vi "Read.vi"(7 "timeout (100ms)":i32=100, 8 "error in (no error)":errorcluster, 9 "Interlock in":bool, 11 "Interlock Bool in":refnum<class "Interlock Bool.lvclass">) -> (0 "error out":errorcluster, 1 "Interlock":bool, 2 "Data out":variant, 3 "Interlock Bool out":refnum<class "Interlock Bool.lvclass">, 4 "IL Action":refnum<class "IL Action.lvclass">[](array[class]))   [LabVIEW 2015, in "Interlocks.lvlib" / "Interlock Bool.lvclass"]
uses:
  Interlock Bool.lvclass
  IL Action/IL Action.lvclass
  Interlock/State Enum.ctl
  Interlock Bool.lvclass/Interlock Bool.ctl
  Interlock/Interlock.lvclass/Interlock.ctl
  Interlock/Interlock.lvclass
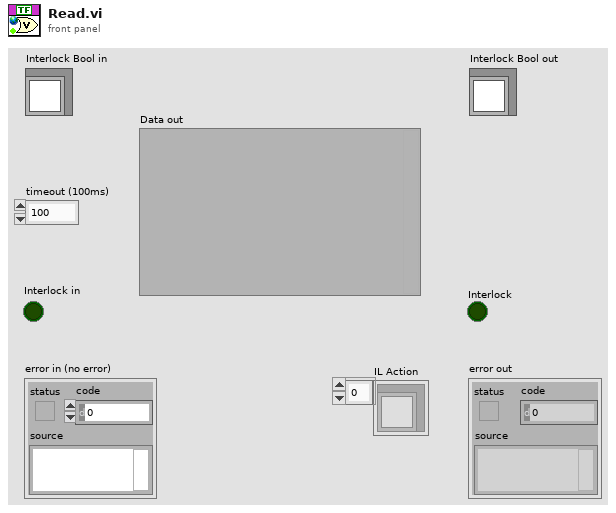
[diagram p1: front panel]
types:
  T1 = typedef "Interlocks.lvlib/Interlock.lvclass/State Enum.ctl" = enum16{"Ok", "Error", "Interlock", "Out of Range", "Is ON", "Is OFF", "Denied", "Not Allowed", "Sample Allow", "Sample Deny"}
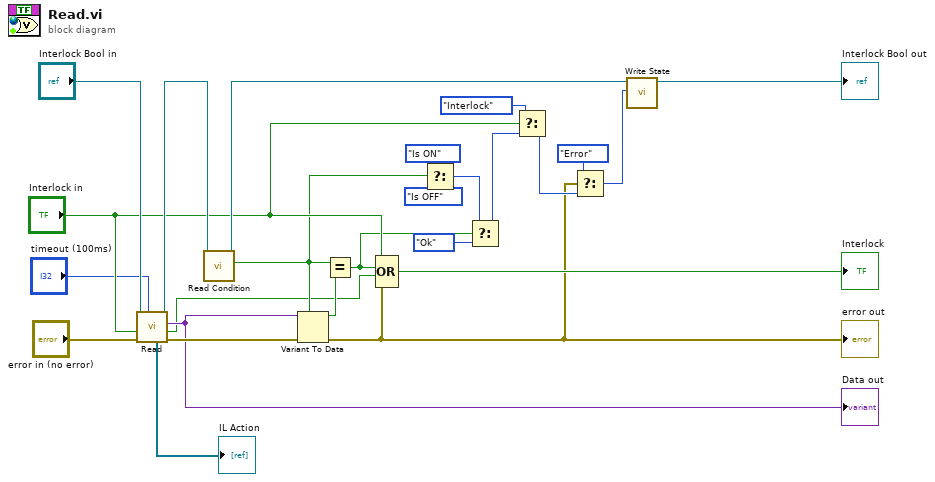
[diagram p0: block diagram]
diagram:
  n1 = call-parent "Read.vi"("timeout (100ms)"="timeout (100ms)", "error in (no error)"="error in (no error)", 9:"Interlock in"="Interlock in", 11:"Interlock in"="Interlock Bool in") -> ("error out"=w21:errorcluster, 1:"Interlock out"=w4:bool, "Data out"=w18:variant, 3:"Interlock out"=w23:refnum<class "Interlock Bool.lvclass">, "IL Action"=→"IL Action":refnum<class "IL Action.lvclass">[])  [unwired: 3 in]
  "Data out" <- w18
  n2 = call "Read Condition.vi"("Interlock Bool in"=w23) -> ("Interlock Condition"=w15:bool, "Interlock Bool out"=w22:refnum<class "Interlock Bool.lvclass">)  [unwired: 9 in]
  n3 = Variant To Data(error in=w21, type=w15, Variant=w18) -> (data=w20:bool, error out=w3:errorcluster)
  "error out" <- w3
  n4 = Equal?(x=w15, y=w20) -> (x = y?=w9:bool)
  n5 = Compound Arithmetic op=OR("Interlock in", w9, w4, w3) -> (→"Interlock":bool)
  n6 = Select(t=State_Enum."Is ON" ("State"), s=w15, f=State_Enum."Is OFF") -> (s? t:f=w13:T1)
  n7 = Select(t=w13, s=w9, f=State_Enum."Ok") -> (s? t:f=w7:T1)
  n8 = Select(t=State_Enum."Interlock" ("State"), s="Interlock in", f=w7) -> (s? t:f=w8:T1)
  n9 = Select(t=State_Enum."Error" ("State"), s=w3, f=w8) -> (s? t:f=w6:T1)
  n10 = call "Write State.vi"("State"=w6, "Interlock in"=w22) -> ("Interlock out"=→"Interlock Bool out":refnum<class "Interlock Bool.lvclass">)  [unwired: 9 in]
